vi "Read Data Xfer.vi"(8 "Error In":errorcluster, 10 "Oldest time to Plot":dbl, 11 "Device Name":string) -> (0 "Error Out":errorcluster, 1 "Latest Timestamp":dbl, 2 "Latest Value":dbl, 3 "Truncated Data History":T1)   [LabVIEW 2014]
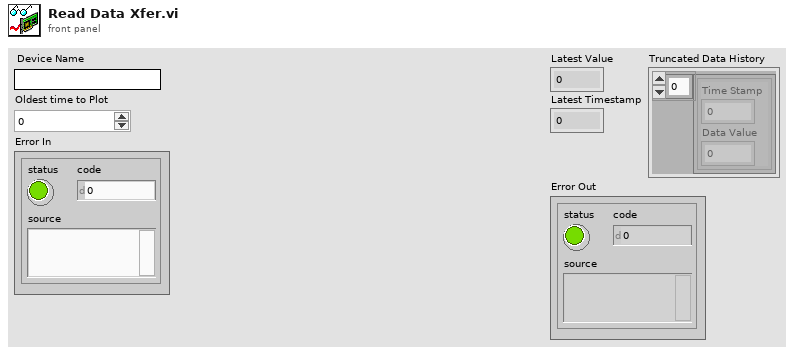
[diagram p1: front panel]
types:
  T1 = cluster{cluster{"Time Stamp":dbl, "Data Value":dbl}[]}
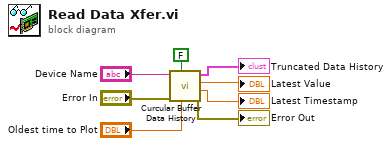
[diagram p0: block diagram]
diagram:
  n1 = call "Curcular Buffer Data History.vi"("Oldest time to Plot"="Oldest time to Plot", "write (F)"=FALSE, "Error In"="Error In", "Device Name"="Device Name") -> ("Error Out"=→"Error Out":errorcluster, "Latest Timestamp"=→"Latest Timestamp":dbl, "Latest Value"=→"Latest Value":dbl, "Truncated Data History"=→"Truncated Data History":T1)  [unwired: 4 in]
